vi "MGI Running Minimum (DBL).vi"(9 "Initialize? (F)":bool, 10 "Size":i32, 11 "Value":dbl format="%.2f") -> (3 "Minimum":dbl format="%.2f")   [LabVIEW 2016]
doc: "Keep a running minimum efficiently.\n\nAuthored by David A Moore\nsupport@mooregoodideas.com\nwww.mooregoodideas.com\n\nCopyright (c) 2010, Moore Good Ideas, Inc.\n\nAll rights reserved.\n\nRedistribution and use in source and binary forms, with or without modification, are permitted provided that the following conditions are met:\n\n * Redistributions of source code must retain the above copyright notice, this list of conditions and the following disclaimer.\n * Redistributions in binary form must reproduce the above copyright notice, this list of conditions and the following disclaimer in the documentation and/or other materials provided with the distribution.\n * Neither the name of Moore Good Ideas, Inc. nor the names of its contributors may be used to endorse or promote products derived from this software without specific prior written permission.\n\nTHIS SOFTWARE IS PROVIDED BY THE COPYRIGHT HOLDERS AND CONTRIBUTORS \"AS IS\" AND ANY EXPRESS OR IMPLIED WARRANTIES, INCLUDING, BUT NOT LIMITED TO, THE IMPLIED WARRANTIES OF MERCHANTABILITY AND FITNESS FOR A PARTICULAR PURPOSE ARE DISCLAIMED. IN NO EVENT SHALL THE COPYRIGHT OWNER OR CONTRIBUTORS BE LIABLE FOR ANY DIRECT, INDIRECT, INCIDENTAL, SPECIAL, EXEMPLARY, OR CONSEQUENTIAL DAMAGES (INCLUDING, BUT NOT LIMITED TO, PROCUREMENT OF SUBSTITUTE GOODS OR SERVICES; LOSS OF USE, DATA, OR PROFITS; OR BUSINESS INTERRUPTION) HOWEVER CAUSED AND ON ANY THEORY OF LIABILITY, WHETHER IN CONTRACT, STRICT LIABILITY, OR TORT (INCLUDING NEGLIGENCE OR OTHERWISE) ARISING IN ANY WAY OUT OF THE USE OF THIS SOFTWARE, EVEN IF ADVISED OF THE POSSIBILITY OF SUCH DAMAGE."
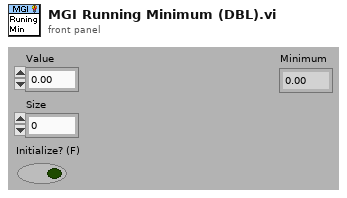
[diagram p1: front panel]
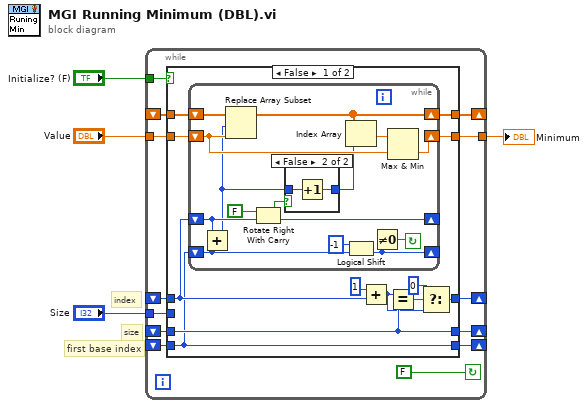
[diagram p0: block diagram]
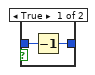
[diagram p2: hidden frame]
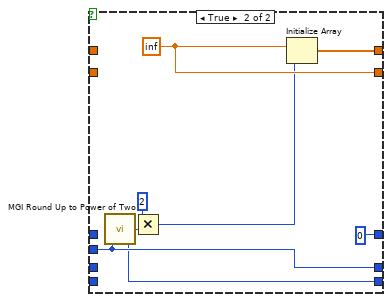
[diagram p3: hidden frame]
diagram:
  # "index"
  # "first base index"
  # "size"
  n1 = while {
    shift-left: _ -> [w5]
    shift-right: [w6] -> _
    tunnel: [w7] -> w1
    tunnel: "Size" -> [w8]
    tunnel: "Value" -> [w9]
    shift-left: _ -> [w10]
    shift-right: [w11] -> _
    tunnel: "Initialize? (F)" -> [w12]
    shift-left: _ -> [w13]
    shift-right: [w16] -> _
    shift-left: _ -> [w14]
    shift-right: [w17] -> _
    stop <- FALSE continue-if-true
    n2 = case shown="False" w12 {
      tunnel: [w22 w55] -> w17
      tunnel: [w29 w52] -> w16
      tunnel: w14 -> [w23 _]
      tunnel: w13 -> [w29 _]
      tunnel: [w26 0 ("Size")] -> w11
      tunnel: w10 -> [w21 _]
      tunnel: w9 -> [w20 _]
      tunnel: w8 -> [_ w52]
      tunnel: [w18 w53] -> w7
      tunnel: [w19 w51] -> w6
      tunnel: w5 -> [w19 _]
      frame False {
        n3 = while {
          shift-left: w19 -> [w43]
          shift-right: [w42] -> _
          shift-left: w20 -> [w36]
          shift-right: [w30] -> w18
          shift-left: w21 -> [w39]
          shift-right: [w38] -> _
          shift-left: w23 -> [w44]
          shift-right: [w35] -> w22
          stop <- w41 continue-if-true
          n4 = Add(x=w39, y=w43) -> (x+y=w32:i32)
          n5 = Replace Array Subset(array=w44, new element=w36, index=w32) -> (w35:dbl[])
          n6 = Rotate Right With Carry(2:w39, 3:FALSE ("carry")) -> (0:w38:i32, 1:w33:bool)
          n7 = case shown="False" w33 {
            tunnel: w32 -> [w46 w48]
            tunnel: [w45 w47] -> w31
            frame True {
              n8 = Decrement(x=w46) -> (x-1=w45:i32)
            }
            frame False {
              n9 = Increment(x=w48) -> (x+1=w47:i32)
            }
          }
          n10 = Index Array(array=w35, index=w31) -> (element=w34:dbl)
          n11 = Logical Shift(y=-1, x=w43) -> (x << y=w42:i32)
          n12 = Not Equal To 0?(x=w42) -> (x != 0?=w41:bool)
          n13 = Max & Min(x=w34, y=w36) -> (min(x,y)=w30:dbl)  [unwired: 1 out]
        }
        n14 = Add(x=1 ("y"), y=w21) -> (x+y=w24:i32)
        n15 = Equal?(x=w24, y=w29) -> (x = y?=w28:bool)
        n16 = Select(t=0, s=w28, f=w24) -> (s? t:f=w26:i32)
      }
      frame True {
        w53 = inf
        n17 = call <userlib>:"MGI Round Up to Power of Two.vi"("Integer"=w52) -> ("Power of 2 Integer"=w51:i32)
        n18 = Multiply(x=2, y=w51) -> (x*y=w49:i32)
        n19 = Initialize Array(w53, w49) -> (w55:dbl[])
      }
    }
  }
  "Minimum" <- w1
